vi "Find term type by ID (type).vi"(7 "Search ID":string, 8 "error in (no error)":errorcluster, 11 "Term Types":T1[](array[typedef])) -> (0 "error out":errorcluster, 1 "Term Type":T1, 2 "index of term":i32, 3 "Other Term Types":T1[](array[typedef]), 5 "Found ?":bool)   [LabVIEW 2018, in "Scripting Tools.lvlib" / "XNode Support.lvlib"]
doc: "Search the <b>term types</b> array for one with the <b>Search ID</b> and return the corresponding <b>Term Type</b>. If found then returns true to <b>Found?</b>."
uses:
  XNode Support.lvlib
  <vilib>/XNodeSupport/XNodeString.ctl
  <vilib>/XNodeSupport/NI_XNodeSupport.lvlib
  <vilib>/XNodeSupport/XNodeType.ctl
  <vilib>/XNodeSupport/XNodeTermTypeIDPair.ctl
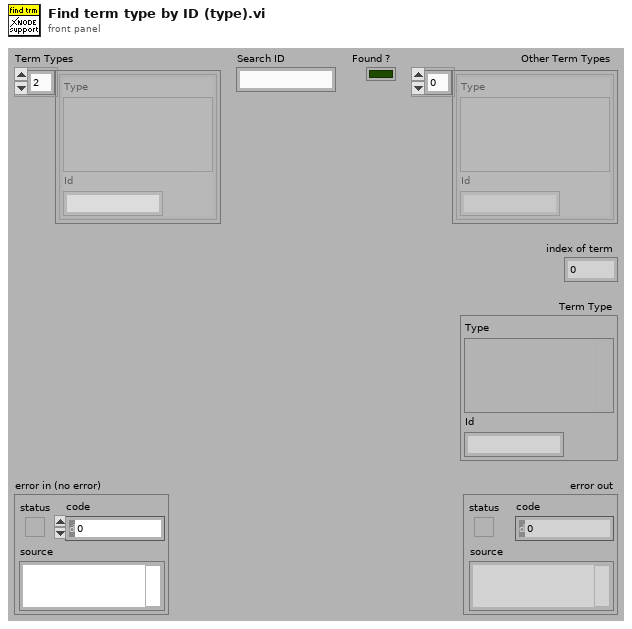
[diagram p1: front panel]
types:
  T1 = typedef "NI_XNodeSupport.lvlib/XNodeTermTypeIDPair.ctl" = cluster{"Type":T2, "Id":T3}
  T2 = typedef "NI_XNodeSupport.lvlib/XNodeType.ctl" = variant
  T3 = typedef "NI_XNodeSupport.lvlib/XNodeString.ctl" = string
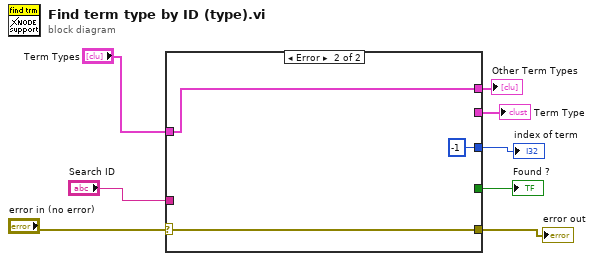
[diagram p0: block diagram]
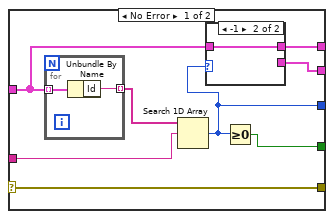
[diagram p2: hidden frame]
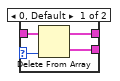
[diagram p3: hidden frame]
diagram:
  n1 = case shown="Error" "error in (no error)" {
    selector: "error in (no error)" -> [w11 w26]
    tunnel: [w11 w26] -> w7
    tunnel: [w14 _] -> w6
    tunnel: [w12 _] -> w5
    tunnel: "Term Types" -> [w13 w24]
    tunnel: "Search ID" -> [w15 _]
    tunnel: [w9 -1 ("index of element")] -> w2
    tunnel: [w10 w24] -> w1
    frame No Error {
      n2 = for {
        tunnel: w13 -> [w23] mode=indexing
        tunnel: [w22] -> w16 mode=indexing
        n3 = Unbundle By Name(w23) -> ("Id"=w22:T3)
      }
      n4 = Search 1D Array(1D array=w16, element=w15) -> (index of element=w9:i32)  [unwired: 1 out]
      n5 = case shown="-1" w9 {
        selector: w9 -> [w17 _]
        tunnel: w13 -> [w20 w21]
        tunnel: [w19 _] -> w12
        tunnel: [w18 w21] -> w10
        frame 0, Default {
          n6 = Delete From Array(array=w20, index=w17) -> (deleted portion=w19:T1, array with subset deleted=w18:T1[])  [unwired: 1 in]
        }
        frame -1 {
        }
      }
      n7 = Greater Or Equal To 0?(x=w9) -> (x >= 0?=w14:bool)
    }
    frame Error {
    }
  }
  "error out" <- w7
  "Term Type" <- w5
  "Found ?" <- w6
  "index of term" <- w2
  "Other Term Types" <- w1
